vi "Close.vi"(8 "error in":errorcluster, 11 "Voltage Nominal Value in":refnum<class "Voltage Nominal Value.lvclass">) -> (0 "error out":errorcluster, 3 "Voltage Nominal Value out":refnum<class "Voltage Nominal Value.lvclass">)   [LabVIEW 2023, in "Voltage Nominal Value.lvclass"]
uses:
  Voltage Nominal Value.lvclass
  Parents/Nominal Value/Nominal Value.lvclass
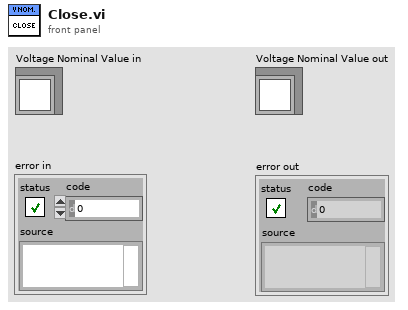
[diagram p1: front panel]
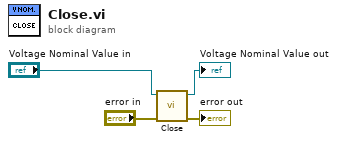
[diagram p0: block diagram]
diagram:
  n1 = call-parent "Close.vi"("error in"="error in", "Nominal Value in"="Voltage Nominal Value in") -> ("error out"=→"error out":errorcluster, "Nominal Value out"=→"Voltage Nominal Value out":refnum<class "Voltage Nominal Value.lvclass">)  [unwired: 8 in]
